vi "Get Output States.vi"(8 "error in (no error)":errorcluster, 11 "VISA resource name":refnum<visa-resource-name>) -> (0 "error out":errorcluster, 2 "Output?":bool, 3 "VISA resource name out":refnum<visa-resource-name>)   [LabVIEW 2014, in "Associated Power Technologies 8500 Series.lvlib"]
doc: "Get the output states of the controlled APT8500."
uses:
  <instrlib>/Associated Power Technologies 8500 Series/Associated Power Technologies 8500 Series.lvlib
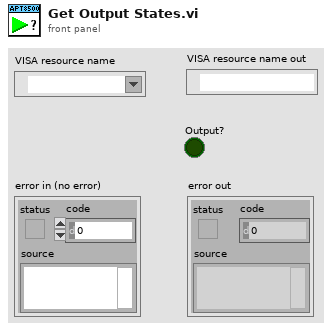
[diagram p1: front panel]
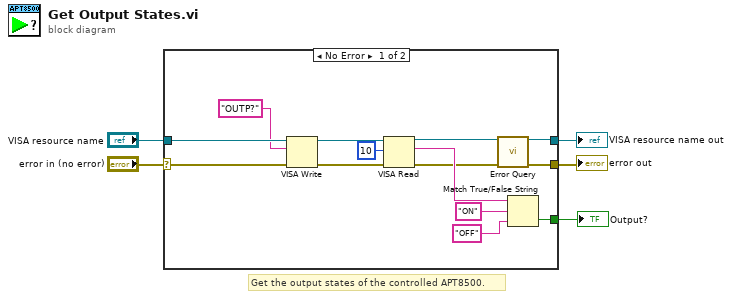
[diagram p0: block diagram]
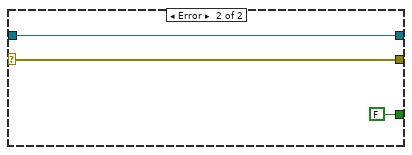
[diagram p2: hidden frame]
diagram:
  # "Get the output states of the controlled APT8500."
  n1 = case shown="No Error" "error in (no error)" {
    selector: "error in (no error)" -> [w18 w21]
    tunnel: "VISA resource name" -> [w19 w22]
    tunnel: [w7 w22] -> w3
    tunnel: [w6 w21] -> w2
    tunnel: [w10 FALSE ("selection")] -> w1
    frame No Error {
      n2 = VISA Write(VISA resource name=w19, write buffer="OUTP?" ("command"), error in (no error)=w18) -> (VISA resource name out=w14:refnum<visa-resource-name>, error out=w17:errorcluster)  [unwired: 1 out]
      n3 = VISA Read(VISA resource name=w14, byte count=u32 10, error in (no error)=w17) -> (VISA resource name out=w9:refnum<visa-resource-name>, read buffer=w13:string, error out=w8:errorcluster)  [unwired: 1 out]
      n4 = call <instrlib>:"Error Query.vi"("VISA resource name"=w9, "error in (no error)"=w8) -> ("VISA resource name out"=w7:refnum<visa-resource-name>, "error out"=w6:errorcluster)  [unwired: 10 in, 2 out]
      n5 = Match True/False String(2:"OFF" ("false string"), 3:"ON" ("true string"), 4:w13) -> (0:w10:bool)  [unwired: 1 out]
    }
    frame Error {
    }
  }
  "VISA resource name out" <- w3
  "error out" <- w2
  "Output?" <- w1
